vi "Read Alarm Limits - Low Warning Limit.vi"(8 "error in (no error)":errorcluster, 11 "NT Scalar (Numeric) in":refnum<class "NT Scalar (Numeric).lvclass">) -> (0 "error out":errorcluster, 2 "low warning limit":dbl format="%.2f", 3 "NT Scalar (Numeric) out":refnum<class "NT Scalar (Numeric).lvclass">)   [LabVIEW 2020, in "PV Access.lvlib" / "PV Data.lvlib" / "NT Scalar (Numeric).lvclass"]
uses:
  NT Scalar (Numeric).lvclass
  NT Scalar (Numeric).lvclass/NT Scalar (Numeric).ctl
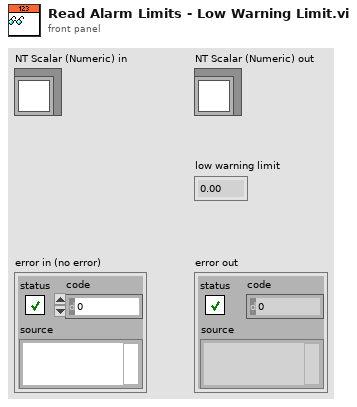
[diagram p1: front panel]
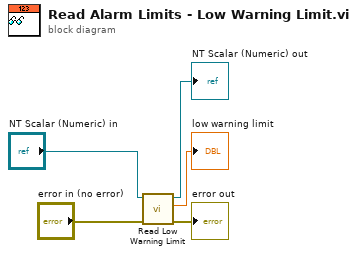
[diagram p0: block diagram]
diagram:
  n1 = call-dynamic "Read Low Warning Limit.vi"("error in"="error in (no error)", "Has Alarm Limits in"="NT Scalar (Numeric) in") -> ("error out"=→"error out":errorcluster, "low warning limit"=→"low warning limit":dbl, "Has Alarm Limits out"=→"NT Scalar (Numeric) out":refnum<class "NT Scalar (Numeric).lvclass">)  [unwired: 7 in]
